vi "Write.vi"(8 "error in (no error)":errorcluster, 9 "Is Raw? (F=Cluster)":bool, 10 "Cluster":variant, 11 "App ID in":u16) -> (0 "error out":errorcluster, 3 "App ID out":u16)   [LabVIEW 2018, in "TCPServer.lvlib"]
uses:
  TCPServer.lvlib
  TypeDefs/CCSDS.ctl
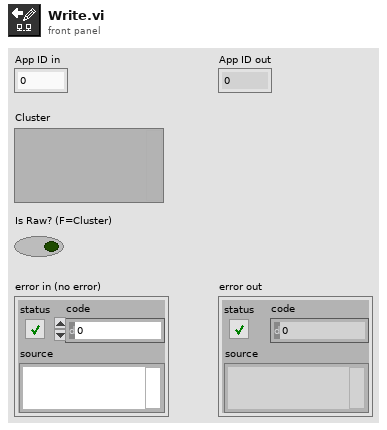
[diagram p1: front panel]
types:
  T1 = typedef "TCPServer.lvlib/CCSDS.ctl" = cluster{"Version":u8, "Type":enum8{"TLM", "CMD"}, "SecHdrFlag":bool, "AppID":u16, "SeqFlags":u8, "SeqCount":u16, "PktLength":u16}
  T2 = typedef "TCPServer.lvlib/App.ctl" = cluster{"Stack":refnum<queue>, "Cmd":cluster{"Conn":refnum<data-value>, "Daemon":refnum<vi>, "Counter":refnum<data-value>}, "Tlm":cluster{"Conn":refnum<data-value>, "Daemon":refnum<vi>, "Counter":refnum<data-value>}}
  T3 = typedef "TCPServer.lvlib/Connection.ctl" = cluster{"Tcp":refnum<k5>, "Server Port":u16, "Server Port Type":enum8{"CMD", "TLM", "BOTH"}, "Client IP":string, "Client Port":u16}
  T4 = typedef "TCPServer.lvlib/Sec Hdr TLM.ctl" = cluster{"DAYS_SINCE_2000":u16, "SECONDS_SINCE_START":u32, "MS_SINCE_START":u16}
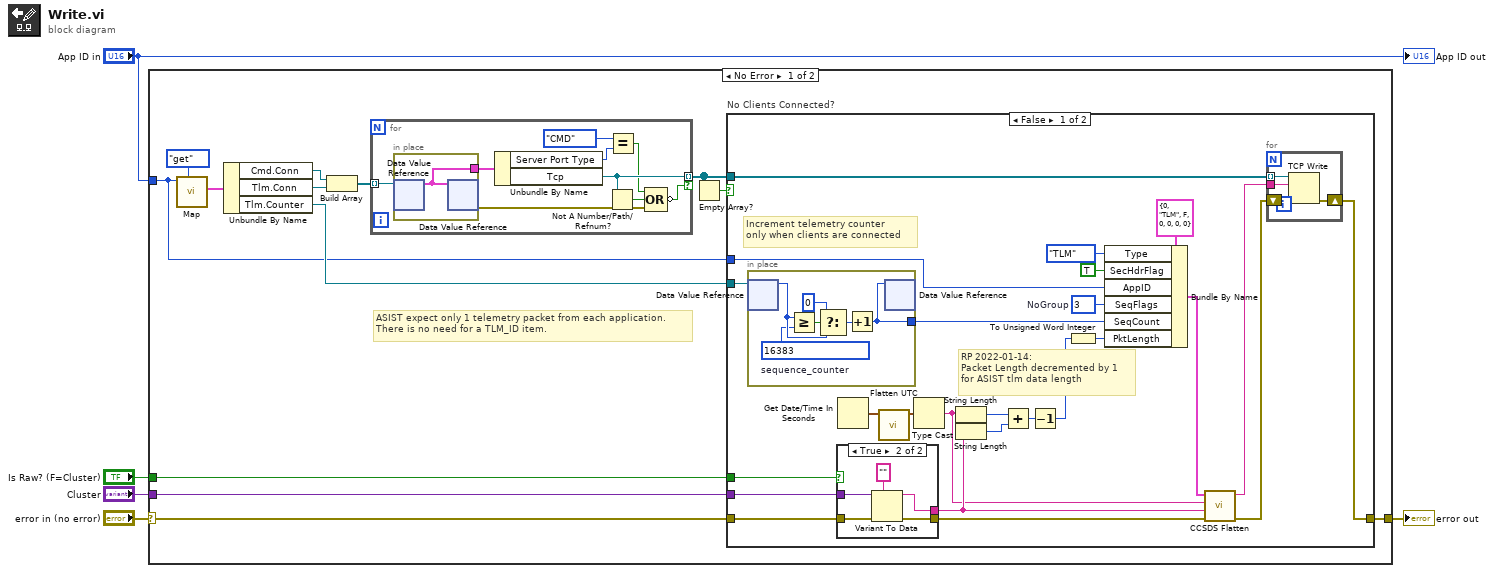
[diagram p0: block diagram]
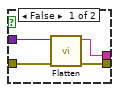
[diagram p2: hidden frame]
diagram:
  n1 = case shown="No Error" "error in (no error)" {
    selector: "error in (no error)" -> [w12 w74]
    tunnel: "Cluster" -> [w17 _]
    tunnel: [w18 w74] -> w3
    tunnel: "Is Raw? (F=Cluster)" -> [w11 _]
    tunnel: "App ID in" -> [w6 _]
    frame No Error {
      # "ASIST expect only 1 telemetry packet from each application.\nThere is no need for a TLM_ID item."
      n2 = call "Map.vi"("Action"=enum8{"noop", "get", "set", "pop"}."get", "App ID in"=w6) -> ("App out"=w9:T2)  [unwired: 7 in, 2 out]
      n3 = Unbundle By Name(w9) -> ("Cmd.Conn"=w7:refnum<data-value>, "Tlm.Conn"=w16:refnum<data-value>, "Tlm.Counter"=w13:refnum<data-value>)
      n4 = Build Array(w7, w16) -> (w8:refnum<data-value>[])
      n5 = for {
        tunnel: w8 -> [w70] mode=indexing
        tunnel: [w68] -> w15 mode=indexing if=w64
        n6 = in-place {
          in-place-border: [w73] -> w69
          n7 = in-place-dvr #1(w70) -> (w73:T3)  [unwired: 1 out]
          n8 = in-place-dvr #1(w73) -> (w66:errorcluster)  [unwired: 1 out]
        }
        n9 = Unbundle By Name(w69) -> ("Server Port Type"=w71:enum8{"CMD", "TLM", "BOTH"}, "Tcp"=w68:refnum<k5>)
        n10 = Not A Number/Path/Refnum?(number/path/refnum=w68) -> (NaN/Path/Refnum?=w67:bool)
        n11 = Equal?(x=enum8{"CMD", "TLM", "BOTH"}."CMD", y=w71) -> (x = y?=w65:bool)
        n12 = Compound Arithmetic op=OR(w65, w67, w66) -> (invert w64:bool)
      }
      n13 = Empty Array?(array=w15) -> (empty?=w14:bool)
      n14 = case "No Clients Connected?" shown="False" w14 {
        tunnel: w15 -> [w43 _]
        tunnel: [w29 w63] -> w18
        tunnel: w12 -> [w23 w63]
        tunnel: w6 -> [w37 _]
        tunnel: w13 -> [w32 _]
        tunnel: w17 -> [w21 _]
        tunnel: w11 -> [w19 _]
        frame False {
          w36 = u8 3  # NoGroup
          # "RP 2022-01-14:\nPacket Length decremented by 1\nfor ASIST tlm data length"
          # "Increment telemetry counter\nonly when clients are connected"
          n15 = in-place {
            in-place-border: [w55] -> w31
            w53 = u16 16383  # sequence_counter
            n16 = in-place-dvr #2(w32) -> (w54:u16)  [unwired: 1 out]
            n17 = Greater Or Equal?(x=w54, y=w53) -> (x >= y?=w58:bool)
            n18 = Select(t=u16 0 ("SeqCount"), s=w58, f=w54) -> (s? t:f=w57:u16)
            n19 = Increment(x=w57) -> (x+1=w55:u16)
            n20 = in-place-dvr #2(w55) -> ()  [unwired: 2 out]
          }
          n21 = case shown="True" w19 {
            tunnel: [w47 w51] -> w24
            tunnel: w23 -> [w46 w52]
            tunnel: [w45 w48] -> w22
            tunnel: w21 -> [w44 w50]
            frame False {
              n22 = call "Flatten.vi"("error in (no error)"=w46, "Cluster"=w44) -> ("error out"=w47:errorcluster, "String"=w45:string)  [unwired: 8 in]
            }
            frame True {
              n23 = Variant To Data(error in=w52, type="", Variant=w50) -> (data=w48:string, error out=w51:errorcluster)
            }
          }
          n24 = Get Date/Time In Seconds() -> (seconds since 1Jan1904=w28:timestamp)
          n25 = call "Flatten UTC.vi"("Local Time in"=w28) -> ("Sec Hdr TLM"=w27:T4)  [unwired: 10 in]
          n26 = Type Cast(x=w27) -> (*(type *) &x=w20:string)  [unwired: 1 in]
          n27 = String Length(string=w20) -> (length=w26:i32)
          n28 = String Length(string=w22) -> (length=w35:i32)
          n29 = Add(x=w26, y=w35) -> (x+y=w34:i32)
          n30 = Decrement(x=w34) -> (x-1=w25:i32)
          n31 = To Unsigned Word Integer(number=w25) -> (unsigned 16bit integer=w33:u16)
          n32 = Bundle By Name(cluster=T1 {"Version"=0, "Type"=enum."TLM", "SecHdrFlag"=FALSE, "AppID"=0, "SeqFlags"=0, "SeqCount"=0, "PktLength"=0} ("CCSDS Primary Header in"), "Type"=enum8{"TLM", "CMD"}."TLM", "SecHdrFlag"=TRUE, "AppID"=w37, "SeqFlags"=w36, "SeqCount"=w31, "PktLength"=w33) -> (w40:T1)
          n33 = call "CCSDS Flatten.vi"("error in (no error)"=w24, "Packet Data in"=w22, "Secondary Header in"=w20, "CCSDS Primary Header in"=w40) -> ("error out"=w30:errorcluster, "CCSDS Packet out"=w41:string)  [unwired: 6 in]
          n34 = for {
            tunnel: w43 -> [w62] mode=indexing
            tunnel: w41 -> [w61]
            shift-right: [w60] -> w29
            shift-left: w30 -> [w59]
            n35 = TCP Write(connection ID=w62, data in=w61, error in (no error)=w59) -> (error out=w60:errorcluster)  [unwired: 1 in, 2 out]
          }
        }
        frame True {
          # "No clients are connected, do nothing."
        }
      }
    }
    frame Error {
    }
  }
  "error out" <- w3
  "App ID out" <- "App ID in"
